vi "test Insert and Delete.vi"(8 "error in (no error)":errorcluster, 11 "TestCase in":refnum<class "Variant Data Manipulation Tests.lvclass">) -> (0 "error out":errorcluster, 3 "TestCase out":refnum<class "Variant Data Manipulation Tests.lvclass">)   [LabVIEW 2017, in "Variant Data Manipulation Tests.lvclass"]
uses:
  Variant Data Manipulation Tests.lvclass
  Source/Insert Element at Start.vi
  Source/Insert Element at End.vi
  Source/Insert Element at Index.vi
  Source/Delete Element at Index.vi
  Source/Delete Last Element.vi
  Source/Delete First Element.vi
  <vilib>/addons/_JKI Toolkits/VI Tester/TestCase.llb/TestCase.lvclass
  Source/Variant Data Manipulation.lvlib
  <vilib>/Utility/Data Type/NI_Data Type.lvlib
  C:/Program Files (x86)/National Instruments/LabVIEW 2017/vi.lib/addons/_JKI Toolkits/VI Tester/TestCase.llb/TestCase.lvclass
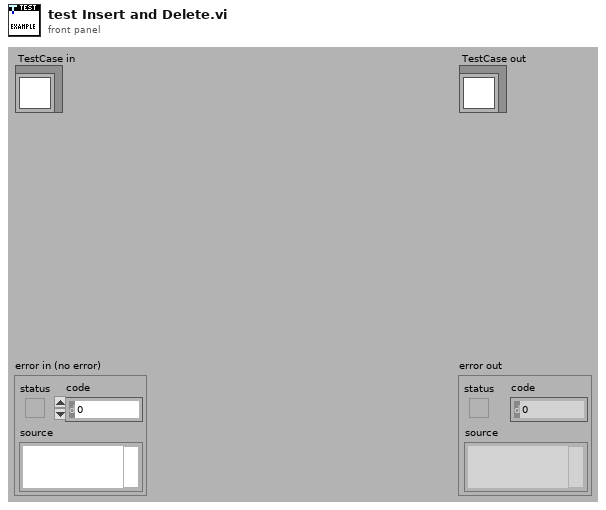
[diagram p1: front panel]
types:
  T1 = cluster{"boolean":bool, "other":string, "string":string, "numeric":i32}
  T2 = cluster{"boolean":bool, "string":string, "numeric":i32}
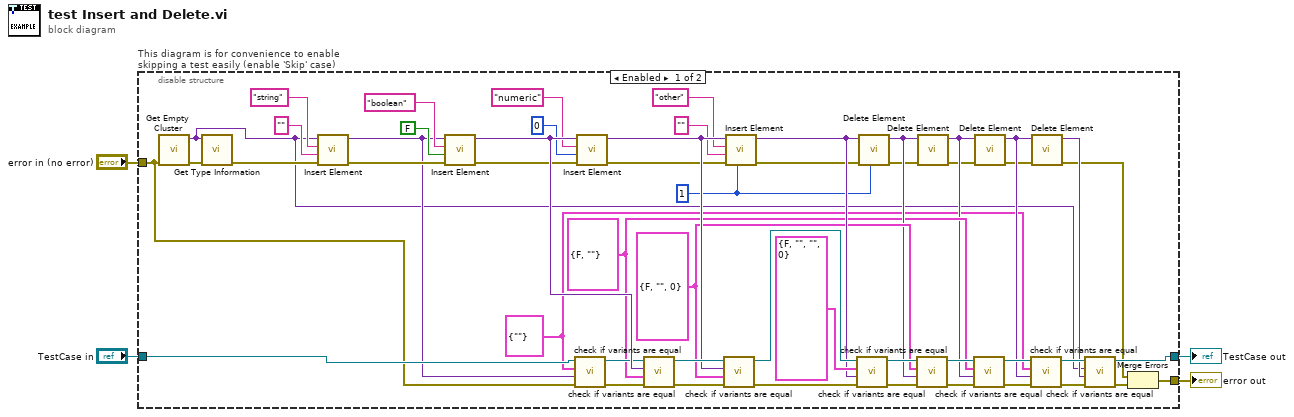
[diagram p0: block diagram]
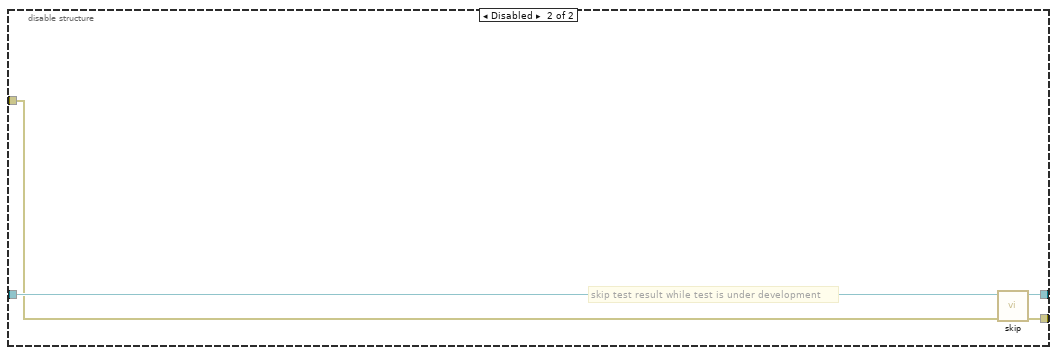
[diagram p2: hidden frame]
diagram:
  n1 = disable-structure "This diagram is for convenience to enable skipping a test easily (enable 'Skip' case)" shown="Enabled" {
    disable-tunnel: "TestCase in" -> [w55 w59]
    disable-tunnel: [w16 w57] -> w1
    disable-tunnel: [w6 w58] -> w3
    disable-tunnel: "error in (no error)" -> [w42 w56]
    frame Enabled {
      w28 = 1 ("index")
      w25 = T2 {"boolean"=FALSE, "string"="", "numeric"=0}
      w21 = cluster{"boolean":bool, "string":string} {"boolean"=FALSE, "string"=""}
      w12 = cluster{"string":string} {"string"=""}
      n2 = call "Get Empty Cluster.vi"("error in (no error)"=w42) -> ("error out"=w54:errorcluster, "Variant (Cluster) out"=w11:variant)  [unwired: 9 in]
      n3 = call <vilib>:"Get Type Information.vi"("error in (no error)"=w54, "Variant"=w11) -> ("error out"=w45:errorcluster)  [unwired: 5 in, 4 out]
      n4 = call-poly "Insert Element.vi"("error in (no error)"=w45, "element"="", "Name"="string", "Variant (Cluster) in"=w11) -> ("error out"=w44:errorcluster, "Variant (Cluster) out"=w30:variant)  [unwired: 6 in]
      n5 = call-poly "Insert Element.vi"("error in (no error)"=w44, "element"=FALSE, "Name"="boolean", "Variant (Cluster) in"=w30) -> ("error out"=w43:errorcluster, "Variant (Cluster) out"=w49:variant)  [unwired: 6 in]
      n6 = call "check if variants are equal.vi"("error in (no error)"=w42, 9:"Variant in"=w30, 10:"Variant in"=w12, "Dynamic Cluster Test in"=w55) -> ("error out"=w32:errorcluster, "Dynamic Cluster Test out"=w31:refnum<class "Variant Data Manipulation Tests.lvclass">)  [unwired: 6 in]
      n7 = call-poly "Insert Element.vi"("error in (no error)"=w43, "element"=0, "Name"="numeric", "Cluster in"=w49) -> ("error out"=w38:errorcluster, "Cluster out"=w39:variant)  [unwired: 6 in]
      n8 = call "check if variants are equal.vi"("error in (no error)"=w32, 9:"Variant in"=w21, 10:"Variant in"=w49, "Dynamic Cluster Test in"=w31) -> ("error out"=w41:errorcluster, "Dynamic Cluster Test out"=w46:refnum<class "Variant Data Manipulation Tests.lvclass">)  [unwired: 6 in]
      n9 = call "check if variants are equal.vi"("error in (no error)"=w41, 9:"Variant in"=w25, 10:"Variant in"=w39, "Dynamic Cluster Test in"=w46) -> ("error out"=w34:errorcluster, "Dynamic Cluster Test out"=w33:refnum<class "Variant Data Manipulation Tests.lvclass">)  [unwired: 6 in]
      n10 = call-poly "Insert Element.vi"("index"=w28, "error in (no error)"=w38, "element"="" ("Name"), "Name"="other", "Cluster in"=w39) -> ("error out"=w10:errorcluster, "Cluster out"=w29:variant)  [unwired: 5 in]
      n11 = call "check if variants are equal.vi"("error in (no error)"=w34, 9:"Variant in"=w29, 10:"Variant in"=T1 {"boolean"=FALSE, "other"="", "string"="", "numeric"=0}, "Dynamic Cluster Test in"=w33) -> ("error out"=w40:errorcluster, "Dynamic Cluster Test out"=w26:refnum<class "Variant Data Manipulation Tests.lvclass">)  [unwired: 6 in]
      n12 = call-poly "Delete Element.vi"("index"=w28, "error in (no error)"=w10, "Cluster in"=w29) -> ("error out"=w9:errorcluster, "Cluster out"=w24:variant)  [unwired: 5 in, 2 out]
      n13 = call "check if variants are equal.vi"("error in (no error)"=w40, 9:"Variant in"=w24, 10:"Variant in"=w25, "Dynamic Cluster Test in"=w26) -> ("error out"=w27:errorcluster, "Dynamic Cluster Test out"=w22:refnum<class "Variant Data Manipulation Tests.lvclass">)  [unwired: 6 in]
      n14 = call-poly "Delete Element.vi"("error in (no error)"=w9, "Cluster in"=w24) -> ("error out"=w8:errorcluster, "Cluster out"=w15:variant)  [unwired: 6 in, 2 out]
      n15 = call "check if variants are equal.vi"("error in (no error)"=w27, 9:"Variant in"=w15, 10:"Variant in"=w21, "Dynamic Cluster Test in"=w22) -> ("error out"=w23:errorcluster, "Dynamic Cluster Test out"=w19:refnum<class "Variant Data Manipulation Tests.lvclass">)  [unwired: 6 in]
      n16 = call-poly "Delete Element.vi"("error in (no error)"=w8, "Cluster in"=w15) -> ("error out"=w7:errorcluster, "Cluster out"=w14:variant)  [unwired: 6 in, 2 out]
      n17 = call "check if variants are equal.vi"("error in (no error)"=w23, 9:"Variant in"=w14, 10:"Variant in"=w12, "Dynamic Cluster Test in"=w19) -> ("error out"=w20:errorcluster, "Dynamic Cluster Test out"=w17:refnum<class "Variant Data Manipulation Tests.lvclass">)  [unwired: 6 in]
      n18 = call-poly "Delete Element.vi"("error in (no error)"=w7, "Cluster in"=w14) -> ("error out"=w5:errorcluster, "Cluster out"=w13:variant)  [unwired: 6 in, 2 out]
      n19 = call "check if variants are equal.vi"("error in (no error)"=w20, 9:"Variant in"=w13, 10:"Variant in"=w11, "Dynamic Cluster Test in"=w17) -> ("error out"=w18:errorcluster, "Dynamic Cluster Test out"=w16:refnum<class "Variant Data Manipulation Tests.lvclass">)  [unwired: 6 in]
      n20 = Merge Errors(w5, w18) -> (w6:errorcluster)
    }
    frame Disabled {
      # "skip test result while test is under development"
      n21 = call <vilib>:"skip.vi"("error in (no error)"=w56, "TestCase in"=w59) -> ("error out"=w58:errorcluster, "TestCase out"=w57:refnum<class "Variant Data Manipulation Tests.lvclass">)  [unwired: 8 in]
    }
  }
  "error out" <- w3
  "TestCase out" <- w1
